vi "Open Door.vi"(8 "error in (no error)":errorcluster, 11 "Doors Opening in":refnum<class "Doors Opening.lvclass">) -> (0 "error out":errorcluster, 3 "Doors Opening out":refnum<class "Doors Opening.lvclass">)   [LabVIEW 2020, in "Door Controller.lvlib" / "Doors Opening.lvclass"]
uses:
  Doors Opening.lvclass
  Doors Opening.lvclass/Doors Opening.ctl
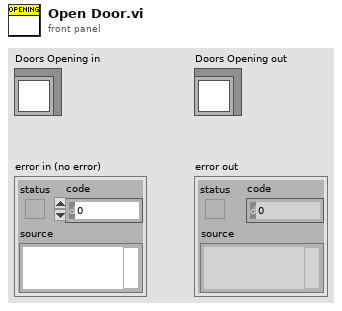
[diagram p1: front panel]
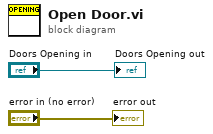
[diagram p0: block diagram]
diagram:
  "error out" <- "error in (no error)"
  "Doors Opening out" <- "Doors Opening in"
